vi "Mutiple String Key To 1D String Array.vi"(7 "Section In":string, 8 "Error In":errorcluster, 10 "Keys In":string[](array[string]), 11 "Ref In":T1) -> (0 "Error Out":errorcluster, 2 "1D String Array Out":string[](array[string]), 3 "Ref Out":T1)   [LabVIEW 2024]
uses:
  <vilib>/Utility/config.llb/Config Data RefNum.ctl
  <vilib>/Utility/config.llb/Read Key (String).vi
  <vilib>/Utility/config.llb/NI_LVConfig.lvlib
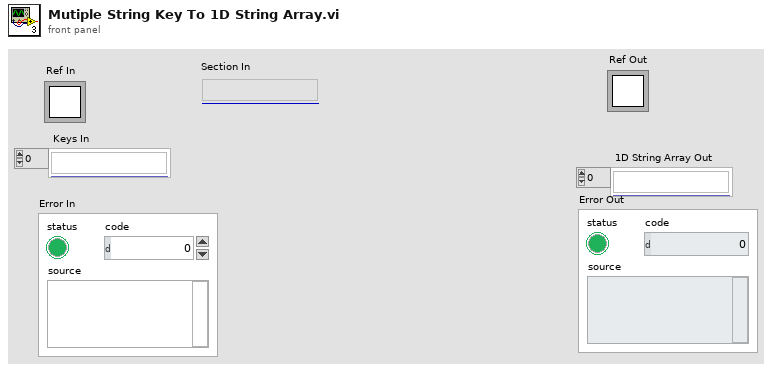
[diagram p1: front panel]
types:
  T1 = typedef "NI_LVConfig.lvlib/Config Data RefNum.ctl" = refnum<k1>
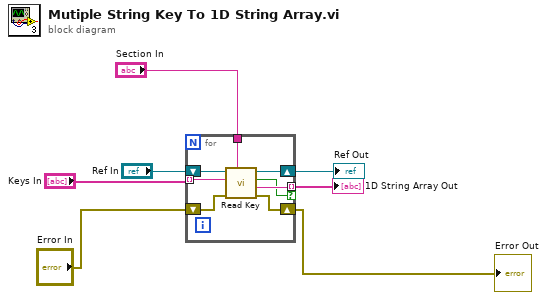
[diagram p0: block diagram]
diagram:
  n1 = for {
    shift-right: [w14] -> w5
    shift-left: "Ref In" -> [w15]
    tunnel: [w13] -> w1 mode=indexing if=w8
    tunnel: "Keys In" -> [w12] mode=indexing
    tunnel: "Section In" -> [w11]
    shift-right: [w9] -> w2
    shift-left: "Error In" -> [w10]
    n2 = call-poly <vilib>:"Read Key.vi"("section"=w11, "error in (no error)"=w10, "key"=w12, "refnum"=w15) -> ("error out"=w9:errorcluster, "value"=w13:string, "found?"=w8:bool, "refnum out"=w14:T1)  [unwired: 4 in]
  }
  "Ref Out" <- w5
  "1D String Array Out" <- w1
  "Error Out" <- w2
